vi "Set Instrument From Marker.vi"(8 "error in (no error)":errorcluster, 9 "Instrument Setting (0: Reference Level)":u16(ring) items=["Reference Level", "Frequency Center", "Frequency Span", "Frequency Start", "Frequency Stop", "Center Frequency Step", "Delta Span", "Delta Center Frequency"], 10 "Active Marker (1: Marker1)":u16(ring)=1 items=["Marker1"=1, "Marker2"=2, "Marker3"=3, "Marker4"=4], 11 "VISA resource name":refnum<visa-resource-name>) -> (0 "error out":errorcluster, 3 "VISA resource name out":refnum<visa-resource-name>)   [LabVIEW 2014, in "Agilent ESA PSA Series.lvlib"]
doc: "Sets the reference level or center frequency to the value of the selected marker."
uses:
  Agilent ESA PSA Series.lvlib
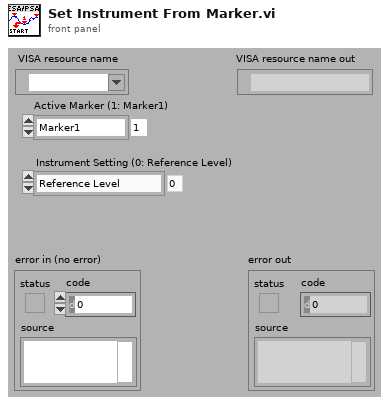
[diagram p1: front panel]
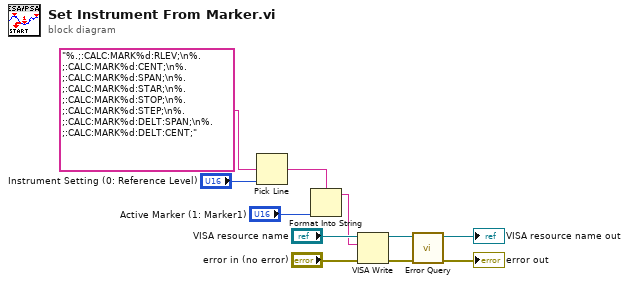
[diagram p0: block diagram]
diagram:
  n1 = Pick Line(multi-line string="%.;:CALC:MARK%d:RLEV;\n%.;:CALC:MARK%d:CENT;\n%.;:CALC:MARK%d:SPAN;\n%.;:CALC:MARK%d:STAR;\n%.;:CALC:MARK%d:STOP;\n%.;:CALC:MARK%d:STEP;\n%.;:CALC:MARK%d:DELT:SPAN;\n%.;:CALC:MARK%d:DELT:CENT;", line index="Instrument Setting (0: Reference Level)") -> (output string=w3:string)  [unwired: 1 in]
  n2 = Format Into String(format string=w3, "Active Marker (1: Marker1)") -> (resulting string=w2:string)  [unwired: 2 in, 1 out]
  n3 = VISA Write(VISA resource name="VISA resource name", write buffer=w2, error in (no error)="error in (no error)") -> (VISA resource name out=w9:refnum<visa-resource-name>, error out=w7:errorcluster)  [unwired: 1 out]
  n4 = call "Error Query.vi"("error in (no error)"=w7, "VISA resource name"=w9) -> ("error out"=→"error out":errorcluster, "VISA resource name out"=→"VISA resource name out":refnum<visa-resource-name>)  [unwired: 6 in, 2 out]
